vi "enum.vi"() -> ()   [LabVIEW 2020]
panel:
  out "selection":string="apple"
  in  "fruit":enum16{"apple", "bananna"}(ring)
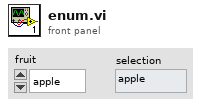
[diagram p1: front panel]
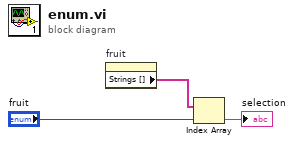
[diagram p0: block diagram]
diagram:
  n1 = property on="fruit" class="Enum (strict)"() -> ("Strings []"=w2:string[])  [unwired: 2 in, 2 out]
  n2 = Index Array(array=w2, index="fruit") -> (element=→"selection":string)
